vi "st_Poisson Inverse CDF (kx).vi"(10 "lambda":dbl=1.0, 11 "cdf(x)":dbl=0.999) -> (0 "error":i32, 3 "x":dbl=4.722291756604139)   [LabVIEW 2010, in "NI_Gmath.lvlib"]
uses:
  NI_Gmath.lvlib
  st_error_code.ctl
panel:
  # "Poisson Inverse CDF"
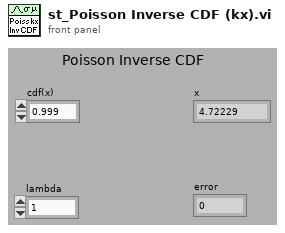
[diagram p1: front panel]
types:
  T1 = typedef "NI_Gmath.lvlib/st_error_code.ctl" = i32
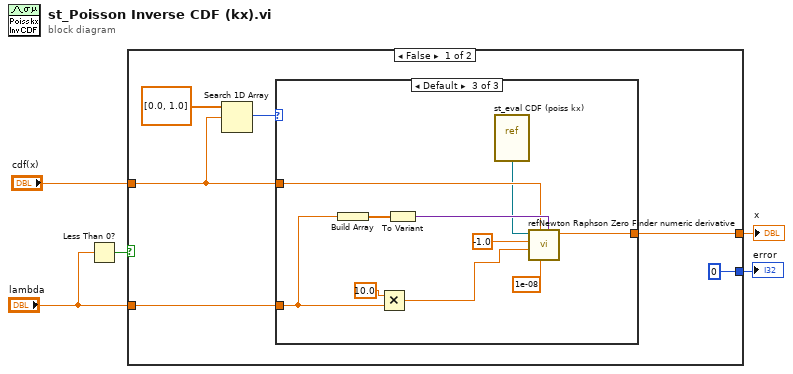
[diagram p0: block diagram]
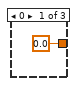
[diagram p2: hidden frame]
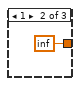
[diagram p3: hidden frame]
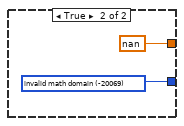
[diagram p4: hidden frame]
diagram:
  n1 = Less Than 0?(x="lambda") -> (x < 0?=w1:bool)
  n2 = case shown="False" w1 {
    tunnel: "lambda" -> [w9 _]
    tunnel: [0 ("invalid math domain") w24] -> w5
    tunnel: [w10 nan] -> w4
    tunnel: "cdf(x)" -> [w6 _]
    frame False {
      n3 = Search 1D Array(1D array=dbl[] [0.0, 1.0], element=w6) -> (index of element=w7:i32)  [unwired: 1 in]
      n4 = case shown="Default" w7 {
        tunnel: [0.0 ("zero") inf ("zero") w22] -> w10
        tunnel: w6 -> [_ _ w20]
        tunnel: w9 -> [_ _ w14]
        frame 0 {
        }
        frame 1 {
        }
        frame Default {
          n5 = Build Array(w14) -> (w23:dbl[])
          n6 = Multiply(x=10.0, y=w14) -> (x*y=w15:dbl)
          n7 = To Variant(anything=w23) -> (Variant=w21:variant)
          n8 = vi-ref "st_eval CDF (poiss kx).vi"() -> ("vi reference"=w19:refnum<vi>)
          n9 = call "refNewton Raphson Zero Finder numeric derivative.vi"("function parameters"=w21, "accuracy"=1e-08, "level"=w20, "end"=w15, "start"=-1.0, "function refnum"=w19) -> ("zero"=w22:dbl)  [unwired: 2 in, 3 out]
        }
      }
    }
    frame True {
      w24 = T1 -20069 items=["invalid math domain"=-20069, "Fourier interpolation size m >= n"=-20070, "empty array"=-20003] ("stat interp error code")
    }
  }
  "x" <- w4
  "error" <- w5
